vi "Core.vi"(8 "error in (no error)":errorcluster, 11 "MB in":refnum<class "WebSocket Client CR.lvclass">) -> (0 "error out":errorcluster, 3 "MB out":refnum<class "WebSocket Client CR.lvclass">)   [LabVIEW 2021, in "WebSockets.lvlib" / "WebSocket Client CR.lvclass"]
uses:
  WebSocket Client CR.lvclass
  ctl/CR_Core_State.ctl
  WebSocket Client CR.lvclass/WebSocket Client CR.ctl
  Status/Run/Write Run.vi
  Status/write/Write write.vi
  Modbus_v121c/Data Model/Device Data Model.lvclass
panel:
  in  "write enable":bool=TRUE
  out "CR_Core_State":T1=enum."requests"
  in  "stop":bool
  out "stopped":bool
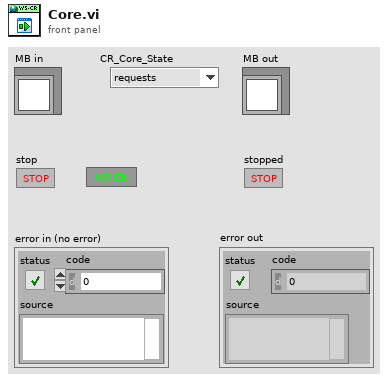
[diagram p1: front panel]
types:
  T1 = typedef "WebSockets.lvlib/WebSocket Client CR.lvclass/CR_Core_State.ctl" = enum8{"initialization", "redefine", "standby", "ping", "connect", "wait to reconnect", "wait to reset timeout", "configure", "requests", "close connection", "stop"}
  T2 = typedef "WebSockets.lvlib/WebSocket Client CR.lvclass/MB timeouts.ctl" = cluster{"reconn_timeout":i32, "N attempt max":i32, "t_reset_TTL":i32, "period":i32}
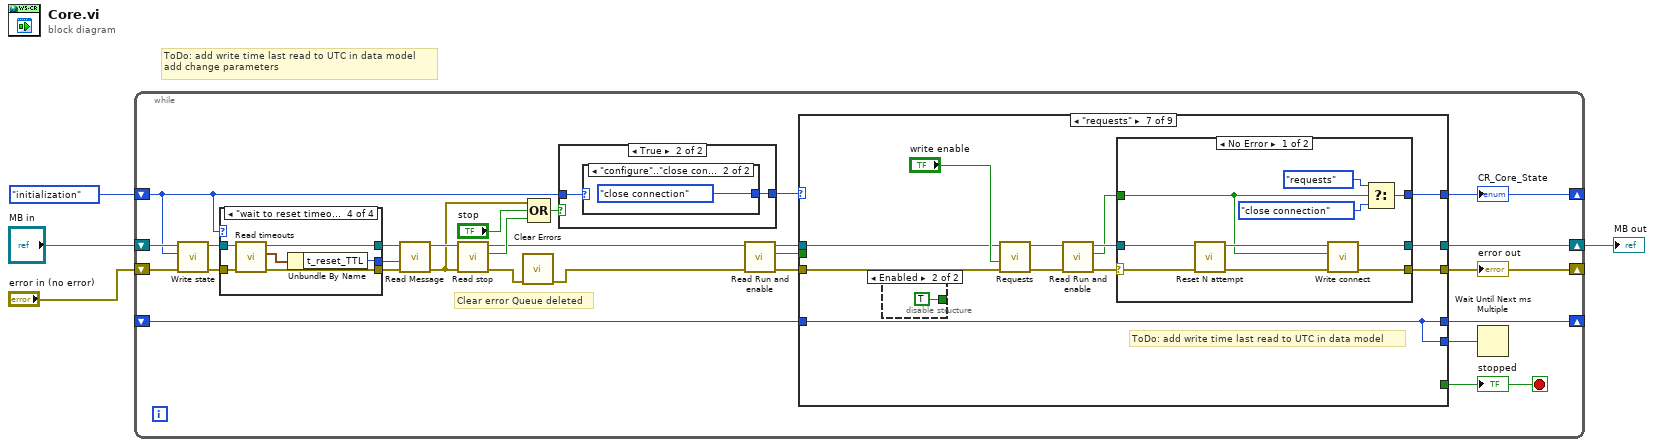
[diagram p0: block diagram]
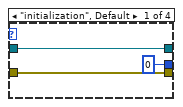
[diagram p2: hidden frame]
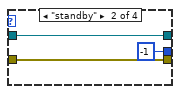
[diagram p3: hidden frame]
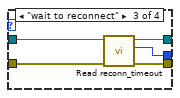
[diagram p4: hidden frame]
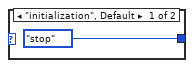
[diagram p6: hidden frame]
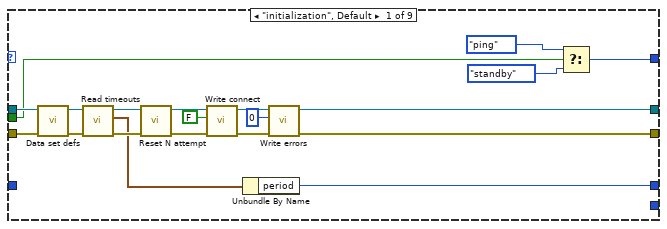
[diagram p7: hidden frame]
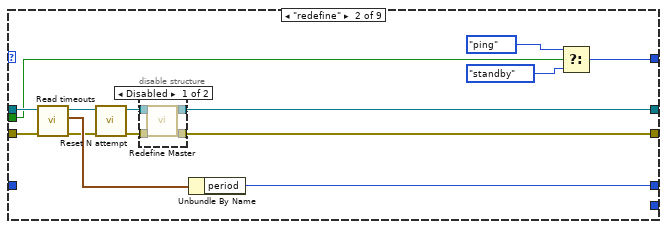
[diagram p8: hidden frame]
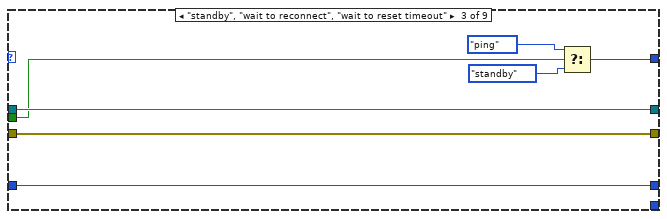
[diagram p10: hidden frame]
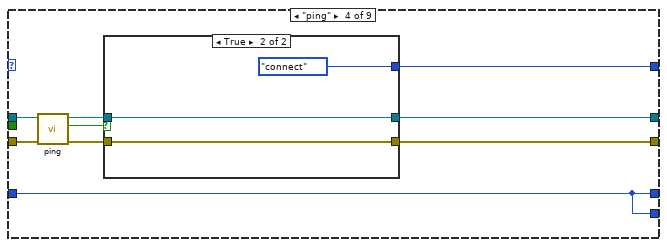
[diagram p11: hidden frame]
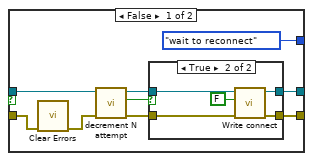
[diagram p12: hidden frame]
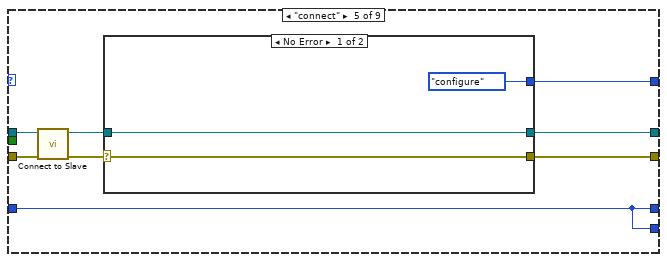
[diagram p14: hidden frame]
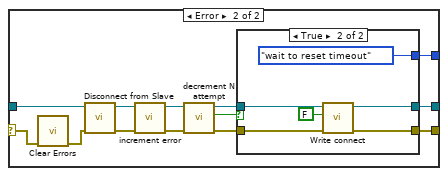
[diagram p15: hidden frame]
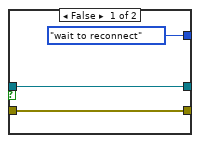
[diagram p16: hidden frame]
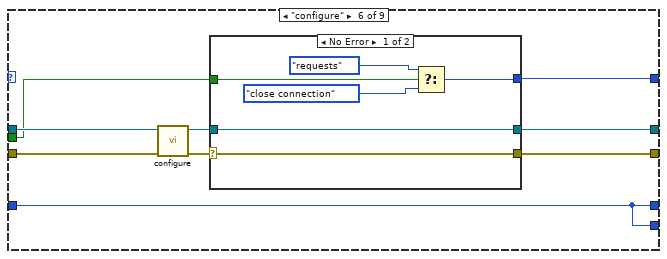
[diagram p17: hidden frame]
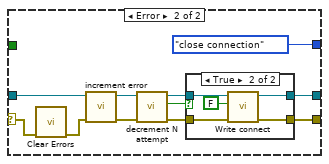
[diagram p18: hidden frame]
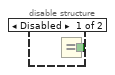
[diagram p20: hidden frame]
diagram:
  # "ToDo: add write time last read to UTC in data model\nadd change parameters"
  n1 = while {
    shift-right: [w28] -> w1
    shift-left: "MB in" -> [w23]
    shift-right: [w13] -> _
    shift-left: "error in (no error)" -> [w22]
    shift-right: [w30] -> _
    shift-left: _ -> [w31]
    shift-right: [w14] -> _
    shift-left: CR_Core_State."initialization" ("state") -> [w19]
    stop <- w12 stop-if-true
    # "Clear error Queue deleted"
    n2 = call "Write state.vi"("error in (no error)"=w22, "state"=w19, "Master CR in"=w23) -> ("error out"=w20:errorcluster, "Master CR out"=w21:refnum<class "WebSocket Client CR.lvclass">)  [unwired: 7 in]
    n3 = case shown="\"wait to reset timeout\"" w19 {
      tunnel: w21 -> [w33 w36 w42 w47]
      tunnel: w20 -> [w32 w35 w41 w46]
      tunnel: [w33 w36 w40 w45] -> w26
      tunnel: [w32 w35 w39 w44] -> w25
      tunnel: [0 ("timeout (0)") -1 ("timeout (0)") w38 w43] -> w24
      frame "initialization", Default {
      }
      frame "standby" {
      }
      frame "wait to reconnect" {
        n4 = call "Read reconn_timeout.vi"("error in (no error)"=w41, "Master CR in"=w42) -> ("error out"=w39:errorcluster, "reconn_timeout"=w38:i32, "Master CR out"=w40:refnum<class "WebSocket Client CR.lvclass">)  [unwired: 7 in]
      }
      frame "wait to reset timeout" {
        n5 = call "Read timeouts.vi"("error in (no error)"=w46, "Master CR in"=w47) -> ("error out"=w44:errorcluster, "MB timeouts"=w48:T2, "Master CR out"=w45:refnum<class "WebSocket Client CR.lvclass">)  [unwired: 7 in]
        n6 = Unbundle By Name(w48) -> ("t_reset_TTL"=w43:i32)
      }
    }
    n7 = call "Read Message.vi"("error in (no error)"=w25, "timeout (0)"=w24, "Master CR in"=w26) -> ("error out"=w11:errorcluster, "Master CR out"=w17:refnum<class "WebSocket Client CR.lvclass">)  [unwired: 6 in, 1 out]
    n8 = call "Read stop.vi"("error in (no error)"=w11, "Master CR in"=w17) -> ("error out"=w15:errorcluster, "Stop"=w16:bool, "Master CR out"=w7:refnum<class "WebSocket Client CR.lvclass">)  [unwired: 7 in]
    n9 = call <vilib>:"Clear Errors.vi"("error in (no error)"=w15) -> ("error out"=w6:errorcluster)  [unwired: 5 in, 1 out]
    n10 = Compound Arithmetic op=OR(w11, "stop", w16) -> (w18:bool)
    n11 = case shown="True" w18 {
      tunnel: w19 -> [w49 w51]
      tunnel: [w49 w50] -> w27
      frame False {
      }
      frame True {
        n12 = case shown="\"configure\"..\"close connection\"" w51 {
          tunnel: [CR_Core_State."stop" ("MB_TCP_State") CR_Core_State."close connection" ("MB_TCP_State")] -> w50
          frame "initialization", Default {
          }
          frame "configure".."close connection" {
          }
        }
      }
    }
    n13 = call "Read Run and enable.vi"("error in (no error)"=w6, "Master CR in"=w7) -> ("error out"=w9:errorcluster, "Enable and Run"=w5:bool, "Master CR out"=w8:refnum<class "WebSocket Client CR.lvclass">)  [unwired: 7 in]
    n14 = case shown="\"requests\"" w27 {
      tunnel: [_ _ _ _ _ _ _ _ TRUE] -> w12
      tunnel: w8 -> [w71 w84 w96 w105 w132 w164 w201 w247 w254]
      tunnel: [w56 w76 w96 w109 w136 w170 w206 w239 w257] -> w28
      tunnel: w9 -> [w72 w83 w95 w104 w133 w163 w200 w246 w253]
      tunnel: [w57 w85 w97 w108 w135 w169 w205 w240 CR_Core_State."initialization" ("MB_TCP_State")] -> w14
      tunnel: [w55 w75 w95 w107 w134 w168 w204 w238 w256] -> w13
      tunnel: [w73 w81 w100 w106 w129 w167 w203 w248 w261] -> w30
      tunnel: w31 -> [_ _ w100 w106 w129 w167 w203 w248 w261]
      tunnel: [_ _ _ w106 w129 w167 w203 _ _] -> w29
      tunnel: w5 -> [w54 w74 w94 _ _ w162 _ w237 _]
      frame "initialization", Default {
        n15 = call "Data set defs.vi"("error in (no error)"=w72, "Master CR in"=w71) -> ("error out"=w66:errorcluster, "Master CR out"=w69:refnum<class "WebSocket Client CR.lvclass">)  [unwired: 8 in]
        n16 = call "Read timeouts.vi"("error in (no error)"=w66, "Master CR in"=w69) -> ("error out"=w70:errorcluster, "MB timeouts"=w67:T2, "Master CR out"=w68:refnum<class "WebSocket Client CR.lvclass">)  [unwired: 7 in]
        n17 = call "Reset N attempt.vi"("error in (no error)"=w70, "Master CR in"=w68) -> ("error out"=w64:errorcluster, "Master CR out"=w65:refnum<class "WebSocket Client CR.lvclass">)  [unwired: 8 in]
        n18 = call "Write connect.vi"("error in (no error)"=w64, "connect"=FALSE, "Master CR in"=w65) -> ("error out"=w62:errorcluster, "Master CR out"=w61:refnum<class "WebSocket Client CR.lvclass">)  [unwired: 7 in]
        n19 = Unbundle By Name(w67) -> ("period"=w73:i32)
        n20 = call "Write errors.vi"("error in (no error)"=w62, "errors"=0, "Master CR in"=w61) -> ("error out"=w55:errorcluster, "Master CR out"=w56:refnum<class "WebSocket Client CR.lvclass">)  [unwired: 7 in]
        n21 = Select(t=CR_Core_State."ping" ("MB_TCP_State"), s=w54, f=CR_Core_State."standby" ("MB_TCP_State")) -> (s? t:f=w57:T1)
      }
      frame "redefine" {
        n22 = call "Read timeouts.vi"("error in (no error)"=w83, "Master CR in"=w84) -> ("error out"=w80:errorcluster, "MB timeouts"=w82:T2, "Master CR out"=w79:refnum<class "WebSocket Client CR.lvclass">)  [unwired: 7 in]
        n23 = call "Reset N attempt.vi"("error in (no error)"=w80, "Master CR in"=w79) -> ("error out"=w77:errorcluster, "Master CR out"=w78:refnum<class "WebSocket Client CR.lvclass">)  [unwired: 8 in]
        n24 = disable-structure shown="Disabled" {
          disable-tunnel: w78 -> [w91 w93]
          disable-tunnel: w77 -> [w90 w92]
          disable-tunnel: [w89 w93] -> w76
          disable-tunnel: [w88 w92] -> w75
          frame Disabled {
            n25 = call "Redefine Master.vi"("error in (no error)"=w90, "Master CR in"=w91) -> ("error out"=w88:errorcluster, "Master CR out"=w89:refnum<class "WebSocket Client CR.lvclass">)  [unwired: 8 in]
          }
          frame Enabled {
          }
        }
        n26 = Unbundle By Name(w82) -> ("period"=w81:i32)
        n27 = Select(t=CR_Core_State."ping" ("MB_TCP_State"), s=w74, f=CR_Core_State."standby" ("MB_TCP_State")) -> (s? t:f=w85:T1)
      }
      frame "standby", "wait to reconnect", "wait to reset timeout" {
        n28 = Select(t=CR_Core_State."ping" ("MB_TCP_State"), s=w94, f=CR_Core_State."standby" ("MB_TCP_State")) -> (s? t:f=w97:T1)
      }
      frame "ping" {
        n29 = call-dynamic "ping.vi"("error in (no error)"=w104, "MB_TCP in"=w105) -> ("error out"=w101:errorcluster, "Ping OK"=w102:bool, "MB_TCP out"=w103:refnum<class "WebSocket Client CR.lvclass">)  [unwired: 7 in]
        n30 = case shown="True" w102 {
          tunnel: w103 -> [w112 w128]
          tunnel: [CR_Core_State."wait to reconnect" ("MB_TCP_State") CR_Core_State."connect" ("MB_TCP_State")] -> w108
          tunnel: [w117 w128] -> w109
          tunnel: [w116 w126] -> w107
          tunnel: w101 -> [w113 w126]
          frame False {
            n31 = call <vilib>:"Clear Errors.vi"("error in (no error)"=w113) -> ("error out"=w111:errorcluster)  [unwired: 5 in, 1 out]
            n32 = call "decrement N attempt.vi"("error in (no error)"=w111, "Master CR in"=w112) -> ("error out"=w114:errorcluster, "=0"=w118:bool, "Master CR out"=w115:refnum<class "WebSocket Client CR.lvclass">)  [unwired: 7 in]
            n33 = case shown="True" w118 {
              tunnel: w115 -> [w120 w122]
              tunnel: [w120 w125] -> w117
              tunnel: w114 -> [w119 w121]
              tunnel: [w119 w123] -> w116
              frame False {
              }
              frame True {
                n34 = call "Write connect.vi"("error in (no error)"=w121, "connect"=FALSE, "Master CR in"=w122) -> ("error out"=w123:errorcluster, "Master CR out"=w125:refnum<class "WebSocket Client CR.lvclass">)  [unwired: 7 in]
              }
            }
          }
          frame True {
          }
        }
      }
      frame "connect" {
        n35 = call-dynamic "Connect to Slave.vi"("error in (no error)"=w133, "network master in"=w132) -> ("error out"=w130:errorcluster, "network master out"=w131:refnum<class "WebSocket Client CR.lvclass">)  [unwired: 8 in]
        n36 = case shown="No Error" w130 {
          selector: w130 -> [w137 w144]
          tunnel: w131 -> [w138 w145]
          tunnel: [CR_Core_State."configure" ("MB_TCP_State") w150] -> w135
          tunnel: [w138 w149] -> w136
          tunnel: [w137 w148] -> w134
          frame No Error {
          }
          frame Error {
            n37 = call <vilib>:"Clear Errors.vi"("error in (no error)"=w144) -> ("error out"=w143:errorcluster)  [unwired: 5 in, 1 out]
            n38 = call-dynamic "Disconnect from Slave.vi"("error in (no error)"=w143, "network master in"=w145) -> ("error out"=w146:errorcluster, "network master out"=w147:refnum<class "WebSocket Client CR.lvclass">)  [unwired: 8 in]
            n39 = call "increment error.vi"("error in (no error)"=w146, "Master CR in"=w147) -> ("error out"=w142:errorcluster, "Master CR out"=w152:refnum<class "WebSocket Client CR.lvclass">)  [unwired: 7 in, 1 out]
            n40 = call "decrement N attempt.vi"("error in (no error)"=w142, "Master CR in"=w152) -> ("error out"=w140:errorcluster, "=0"=w151:bool, "Master CR out"=w141:refnum<class "WebSocket Client CR.lvclass">)  [unwired: 7 in]
            n41 = case shown="True" w151 {
              tunnel: [CR_Core_State."wait to reconnect" ("MB_TCP_State") CR_Core_State."wait to reset timeout" ("MB_TCP_State")] -> w150
              tunnel: w141 -> [w154 w157]
              tunnel: [w154 w160] -> w149
              tunnel: w140 -> [w153 w156]
              tunnel: [w153 w158] -> w148
              frame False {
              }
              frame True {
                n42 = call "Write connect.vi"("error in (no error)"=w156, "connect"=FALSE, "Master CR in"=w157) -> ("error out"=w158:errorcluster, "Master CR out"=w160:refnum<class "WebSocket Client CR.lvclass">)  [unwired: 7 in]
              }
            }
          }
        }
      }
      frame "configure" {
        n43 = call-dynamic "configure.vi"("error in (no error)"=w163, "Master CR in"=w164) -> ("error out"=w165:errorcluster, "Master CR out"=w166:refnum<class "WebSocket Client CR.lvclass">)  [unwired: 8 in]
        n44 = case shown="No Error" w165 {
          selector: w165 -> [w172 w186]
          tunnel: [w176 CR_Core_State."close connection" ("MB_TCP_State")] -> w169
          tunnel: [w172 w179] -> w168
          tunnel: w166 -> [w173 w178]
          tunnel: [w173 w180] -> w170
          tunnel: w162 -> [w171 _]
          frame No Error {
            n45 = Select(t=CR_Core_State."requests" ("MB_TCP_State"), s=w171, f=CR_Core_State."close connection" ("MB_TCP_State")) -> (s? t:f=w176:T1)
          }
          frame Error {
            n46 = call <vilib>:"Clear Errors.vi"("error in (no error)"=w186) -> ("error out"=w177:errorcluster)  [unwired: 5 in, 1 out]
            n47 = call "increment error.vi"("error in (no error)"=w177, "Master CR in"=w178) -> ("error out"=w182:errorcluster, "Master CR out"=w181:refnum<class "WebSocket Client CR.lvclass">)  [unwired: 7 in, 1 out]
            n48 = call "decrement N attempt.vi"("error in (no error)"=w182, "Master CR in"=w181) -> ("error out"=w183:errorcluster, "=0"=w185:bool, "Master CR out"=w184:refnum<class "WebSocket Client CR.lvclass">)  [unwired: 7 in]
            n49 = case shown="True" w185 {
              tunnel: w184 -> [w189 w194]
              tunnel: [w189 w193] -> w180
              tunnel: w183 -> [w188 w192]
              tunnel: [w188 w190] -> w179
              frame False {
              }
              frame True {
                n50 = call "Write connect.vi"("error in (no error)"=w192, "connect"=FALSE, "Master CR in"=w194) -> ("error out"=w190:errorcluster, "Master CR out"=w193:refnum<class "WebSocket Client CR.lvclass">)  [unwired: 7 in]
              }
            }
          }
        }
      }
      frame "requests" {
        # "ToDo: add write time last read to UTC in data model"
        n51 = disable-structure shown="Enabled" {
          disable-tunnel: [w207 TRUE] -> _
          frame Disabled {
            n52 = Equal?() -> (x = y?=w207:bool)  [unwired: 2 in]
          }
          frame Enabled {
          }
        }
        n53 = call-dynamic "Requests.vi"("error in (no error)"=w200, "write enable"="write enable", "TCP Client in"=w201) -> ("error out"=w199:errorcluster, "MB_TCP out"=w197:refnum<class "WebSocket Client CR.lvclass">)  [unwired: 7 in]
        n54 = call "Read Run and enable.vi"("error in (no error)"=w199, "Master CR in"=w197) -> ("error out"=w198:errorcluster, "Enable and Run"=w195:bool, "Master CR out"=w196:refnum<class "WebSocket Client CR.lvclass">)  [unwired: 7 in]
        n55 = case shown="No Error" w198 {
          selector: w198 -> [w214 w229]
          tunnel: [w218 CR_Core_State."close connection" ("MB_TCP_State")] -> w205
          tunnel: w195 -> [w211 _]
          tunnel: [w209 w225] -> w204
          tunnel: w196 -> [w215 w222]
          tunnel: [w212 w226] -> w206
          frame No Error {
            n56 = call "Reset N attempt.vi"("error in (no error)"=w214, "Master CR in"=w215) -> ("error out"=w210:errorcluster, "Master CR out"=w213:refnum<class "WebSocket Client CR.lvclass">)  [unwired: 8 in]
            n57 = call "Write connect.vi"("error in (no error)"=w210, "connect"=w211, "Master CR in"=w213) -> ("error out"=w209:errorcluster, "Master CR out"=w212:refnum<class "WebSocket Client CR.lvclass">)  [unwired: 7 in]
            n58 = Select(t=CR_Core_State."requests" ("MB_TCP_State"), s=w211, f=CR_Core_State."close connection" ("MB_TCP_State")) -> (s? t:f=w218:T1)
          }
          frame Error {
            # "clear read error"
            n59 = call <vilib>:"Clear Errors.vi"("error in (no error)"=w229) -> ("error out"=w221:errorcluster)  [unwired: 5 in, 1 out]
            n60 = call "increment error.vi"("error in (no error)"=w221, "Master CR in"=w222) -> ("error out"=w223:errorcluster, "Master CR out"=w228:refnum<class "WebSocket Client CR.lvclass">)  [unwired: 7 in, 1 out]
            n61 = call "decrement N attempt.vi"("error in (no error)"=w223, "Master CR in"=w228) -> ("error out"=w224:errorcluster, "=0"=w220:bool, "Master CR out"=w227:refnum<class "WebSocket Client CR.lvclass">)  [unwired: 7 in]
            n62 = case shown="False" w220 {
              tunnel: w227 -> [w231 w236]
              tunnel: [w231 w235] -> w226
              tunnel: w224 -> [w230 w234]
              tunnel: [w230 w232] -> w225
              frame False {
              }
              frame True {
                n63 = call "Write connect.vi"("error in (no error)"=w234, "connect"=FALSE, "Master CR in"=w236) -> ("error out"=w232:errorcluster, "Master CR out"=w235:refnum<class "WebSocket Client CR.lvclass">)  [unwired: 7 in]
              }
            }
          }
        }
      }
      frame "close connection" {
        n64 = call-dynamic "Disconnect from Slave.vi"("error in (no error)"=w246, "network master in"=w247) -> ("error out"=w238:errorcluster, "network master out"=w239:refnum<class "WebSocket Client CR.lvclass">)  [unwired: 8 in]
        n65 = disable-structure shown="Enabled" {
          disable-tunnel: [w249 TRUE] -> w241
          frame Disabled {
            n66 = Equal?() -> (x = y?=w249:bool)  [unwired: 2 in]
          }
          frame Enabled {
          }
        }
        n67 = Select(t=CR_Core_State."wait to reconnect" ("MB_TCP_State"), s=w241, f=CR_Core_State."redefine" ("MB_TCP_State")) -> (s? t:f=w243:T1)
        n68 = Select(t=w243, s=w237, f=CR_Core_State."standby" ("MB_TCP_State")) -> (s? t:f=w240:T1)
      }
      frame "stop" {
        n69 = call "Write connect.vi"("error in (no error)"=w253, "connect"=FALSE, "Master CR in"=w254) -> ("error out"=w252:errorcluster, "Master CR out"=w251:refnum<class "WebSocket Client CR.lvclass">)  [unwired: 7 in]
        n70 = call "Write stop.vi"("error in (no error)"=w252, "Stop"=FALSE, "Master CR in"=w251) -> ("error out"=w256:errorcluster, "Master CR out"=w257:refnum<class "WebSocket Client CR.lvclass">)  [unwired: 7 in]
      }
    }
    "CR_Core_State" <- w14
    "error out" <- w13
    "stopped" <- w12
    n71 = Wait Until Next ms Multiple(millisecond multiple=w29) -> ()  [unwired: 1 out]
  }
  "MB out" <- w1
